vi "cRIO_4DoF_vectorcompensation_eightplus.vi"(4 "F_2":dbl[](array[numeric]), 7 "Radius":dbl, 9 "op-space pos\n(global frame)":dbl[](array[numeric]), 10 "Loop_R":bool, 11 "Loop_L":bool) -> (3 "delPosout":dbl[](array[numeric]))   [LabVIEW 2019]
uses:
  <vilib>/imath/engines/lvmath2/RunTimeEngine/IndexRead/NIMS V(R2).vi
  <instcachedir>/0/NIMS V(R2)_C76619605A0E4E9F8B2FA9389712AC47.lvgen/NIMS V(R2)_C76619605A0E4E9F8B2FA9389712AC47_000.vi
  <vilib>/imathl/engines/lvmath/Functions/Error Handling/Create Error.vi
  <vilib>/imath/engines/lvmath2/RunTimeEngine/BuiltInFunctions/all/NIMS_all(GS).vi
  <vilib>/imath/engines/lvmath2/RunTimeEngine/IndexRead/NIMS V(S).vi
  <instcachedir>/0/NIMS V(S)_0488751826AF41519A22953C041130DC.lvgen/NIMS V(S)_0488751826AF41519A22953C041130DC_000.vi
  <vilib>/imath/engines/lvmath2/RunTimeEngine/IndexReplace/NIMS V(S)=S.vi
  <instcachedir>/0/NIMS V(S)=S_BD5C8CB81B6E4D99B8C0034EA1BEE55D.lvgen/NIMS V(S)=S_BD5C8CB81B6E4D99B8C0034EA1BEE55D_000.vi
  <vilib>/imath/engines/lvmath2/RunTimeEngine/ErrorHandling/NIMS_Create Error From Enums.vi
  <vilib>/imath/engines/lvmath2/RunTimeEngine/ArithmeticOperatorToken/NIMS_ArithmeticOperator_power(S).vi
  <instcachedir>/0/NIMS_ArithmeticOperator_power(S)_F1497A2DE3CE4E82B2C3646D59904248.lvgen/NIMS_ArithmeticOperator_power(S)_F1497A2DE3CE4E82B2C3646D59904248_014.vi
  <vilib>/imath/engines/lvmath2/RunTimeEngine/IndexReplace/NIMS V(R2)=V.vi
  <instcachedir>/0/NIMS V(R2)=V_68511C8AEC974C318C65DE7AF205D05C.lvgen/NIMS V(R2)=V_68511C8AEC974C318C65DE7AF205D05C_001.vi
  <vilib>/imath/engines/lvmath2/RunTimeEngine/NodeEndStatement/NIMS_NodeEndStatement_Output.vi
  <instcachedir>/0/NIMS_NodeEndStatement_Output_53EC0D466D134D7ABD903AC30B43404B.lvgen/NIMS_NodeEndStatement_Output_53EC0D466D134D7ABD903AC30B43404B_005.vi
  <vilib>/imath/engines/lvmath2/RunTimeEngine/ErrorHandling/NIMS_Finalize Error.vi
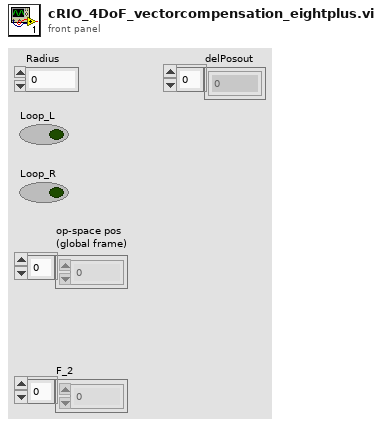
[diagram p1: front panel]
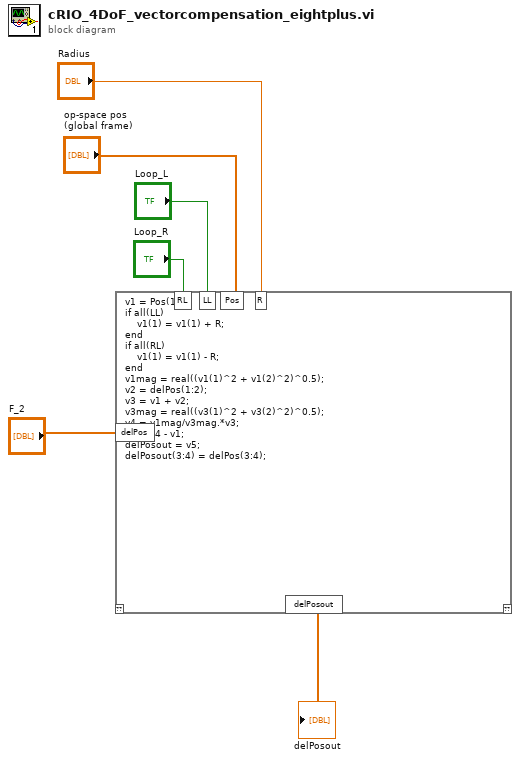
[diagram p0: block diagram]
diagram:
  n1 = mathscript code="v1 = Pos(1:2);\nif all(LL) \n    v1(1) = v1(1) + R;\nend\nif all(RL)\n    v1(1) = v1(1) - R;\nend\nv1mag = real((v1(1)^2 + v1(2)^2)^0.5);\nv2 = delPos(1:2);\nv3 = v1 + v2;\nv3mag = real((v3(1)^2 + v3(2)^2)^0.5);\nv4 = v1mag/v3mag.*v3;\nv5 = v4 - v1;\ndelPosout = v5;\ndelPosout(3:4) = delPos(3:4);"("R"="Radius", "Pos"="op-space pos\n(global frame)", "LL"="Loop_L", "RL"="Loop_R", "delPos"="F_2") -> ("delPosout"=→"delPosout":dbl[])  [unwired: 1 in, 1 out]
